vi "export example information.vi"() -> ()   [LabVIEW 2020]
uses:
  <vilib>/JDP Science/JSONtext/LVClass Serializer/JSONtext LVClass Serializer.lvclass
  4edb9a30-9a21-4ee1-8258-10869d222808.vi
  <vilib>/Utility/NIReport.llb/NI_ReportGenerationCore.lvlib
panel:
  out "error out":errorcluster
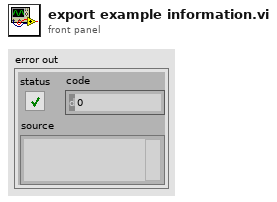
[diagram p1: front panel]
types:
  T1 = enum16{"open", "replace", "create", "open or create", "replace or create", "replace or create with confirmation"}
  T2 = cluster{"Printing:Custom All Controls?":bool, "Printing:Custom Connector?":bool, "Printing:Custom Control Descriptions?":bool, "Printing:Custom Control Types?":bool, "Printing:Custom Controls?":bool, "Printing:Custom Description?":bool, "Printing:Custom Diagram Hidden?":bool, "Printing:Custom Diagram Repeat?":bool, "Printing:Custom Diagram?":bool, "Printing:Custom Hierarchy?":bool, "Printing:Custom History?":bool, "Printing:Custom Panel Border?":bool, "Printing:Custom Panel?":bool, "Printing:Custom SubVIs?":bool}
  T3 = cluster{"vi name":string, "diagram image":path, "description":string}
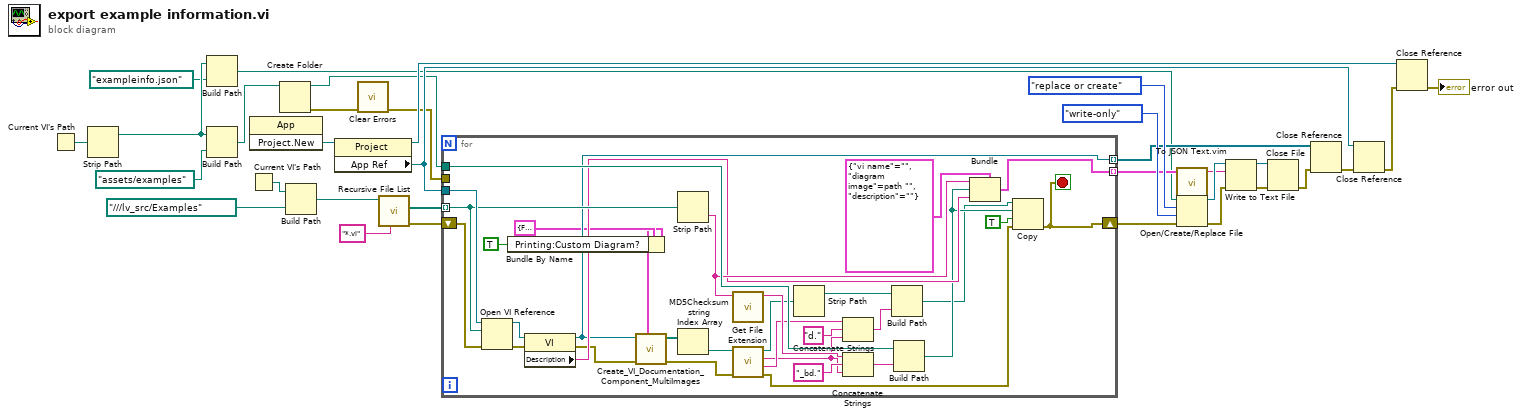
[diagram p0: block diagram]
diagram:
  n1 = Current VI's Path() -> (path=w30:path)
  n2 = Strip Path(path=w30) -> (stripped path=w3:path)  [unwired: 1 out]
  n3 = Build Path(base path=w3, name or relative path=path "exampleinfo.json") -> (appended path=w1:path)
  n4 = Build Path(base path=w3, name or relative path=path "assets/examples") -> (appended path=w9:path)
  n5 = Current VI's Path() -> (path=w32:path)
  n6 = invoke class="App" method="Project.New"() -> ("Project:New"=w25:refnum<vi>)  [unwired: 3 in, 2 out]
  n7 = Create Folder(path (use dialog)=w9) -> (created path=w7:path, error out=w28:errorcluster)  [unwired: 2 in, 1 out]
  n8 = Build Path(base path=w32, name or relative path=path "../../../lv_src/Examples") -> (appended path=w27:path)
  n9 = property class="Project"(reference=w25) -> (reference out=w22:refnum<vi>, "App Ref"=w20:refnum<vi>)  [unwired: 1 in, 1 out]
  n10 = call <vilib>:"Clear Errors.vi"("error in (no error)"=w28) -> ("error out"=w8:errorcluster)  [unwired: 5 in, 1 out]
  n11 = call <vilib>:"Recursive File List.vi"("pattern"="*.vi", "Folder Path"=w27) -> ("error out"=w6:errorcluster, "All Files in Dir"=w19:path[])  [unwired: 5 in, 3 out]
  n12 = for {
    tunnel: w20 -> [w64]
    tunnel: w19 -> [w62] mode=indexing
    tunnel: [w51] -> w10 mode=indexing
    tunnel: w8 -> [_]
    tunnel: w7 -> [w61]
    shift-right: [w37] -> w5
    shift-left: w6 -> [w58]
    tunnel: [w53] -> w4 mode=indexing
    stop <- w37 stop-if-true
    n13 = Open VI Reference(application reference (local)=w64, vi path=w62, error in (no error)=w58) -> (vi reference=w55:refnum<vi>, error out=w63:errorcluster)  [unwired: 3 in]
    n14 = Bundle By Name(cluster=T2 {"Printing:Custom All Controls?"=FALSE, "Printing:Custom Connector?"=FALSE, "Printing:Custom Control Descriptions?"=FALSE, "Printing:Custom Control Types?"=FALSE, "Printing:Custom Controls?"=FALSE, "Printing:Custom Description?"=FALSE, "Printing:Custom Diagram Hidden?"=FALSE, "Printing:Custom Diagram Repeat?"=FALSE, "Printing:Custom Diagram?"=TRUE, "Printing:Custom Hierarchy?"=FALSE, "Printing:Custom History?"=FALSE, "Printing:Custom Panel Border?"=FALSE, "Printing:Custom Panel?"=FALSE, "Printing:Custom SubVIs?"=FALSE} ("Content Options"), "Printing:Custom Diagram?"=TRUE) -> (w34:T2)
    n15 = property class="VI"(reference=w55, error in=w63) -> (reference out=w51:refnum<vi>, error out=w50:errorcluster, "Description"=w54:string)
    n16 = call <vilib>:"Create_VI_Documentation_Component_MultiImages.vi"("Content Options"=w34, "error in (no error)"=w50, "VI"=w51) -> ("error out"=w49:errorcluster, "Paths to images"=w47:path[])  [unwired: 7 in]
    n17 = Strip Path(path=w62) -> (name=w56:string)  [unwired: 1 out]
    n18 = Index Array(array=w47) -> (element=w43:path)  [unwired: 1 in]
    n19 = call "MD5Checksum string.vi"("Message String"=w56) -> ("MD5 message-digest"=w60:string)  [unwired: 10 in]
    n20 = call <vilib>:"Get File Extension.vi"("error in (no error)"=w49, "file"=w43) -> ("error out"=w44:errorcluster, "filename without extension"=w36:string, "lowercase file extension"=w35:string, "dup file"=w42:path)  [unwired: 5 in, 1 out]
    n21 = Strip Path(path=w42) -> (stripped path=w41:path)  [unwired: 1 out]
    n22 = Concatenate Strings(w36, "d." ("string"), w35) -> (w38:string)
    n23 = Concatenate Strings(w60, "_bd." ("string"), w35) -> (w59:string)
    n24 = Build Path(base path=w41, name or relative path=w38) -> (appended path=w40:path)
    n25 = Build Path(base path=w61, name or relative path=w59) -> (appended path=w46:path)
    n26 = Bundle(cluster=T3 {"vi name"="", "diagram image"=path "", "description"=""}, "vi name"=w56, "diagram image"=w46, "description"=w54) -> (w53:T3)
    n27 = Copy(8:w44, 9:TRUE ("overwrite (F)"), 10:w46, 11:w40) -> (0:w37:errorcluster)  [unwired: 1 in, 2 out]
  }
  n28 = call "To JSON Text.vim"("Anything"=w4) -> ("<JSON>"=w12:string)  [unwired: 9 in, 1 out]
  n29 = Open/Create/Replace File(file path (use dialog)=w1, error in=w5, operation (0:open)=T1."replace or create", access (0:read/write)=enum16{"read/write", "read-only", "write-only"}."write-only") -> (refnum out=w15:refnum<file>, error out=w16:errorcluster)  [unwired: 2 in, 1 out]
  n30 = Write to Text File(file (use dialog)=w15, text=w12, error in=w16) -> (refnum out=w17:refnum<file>, error out=w18:errorcluster)  [unwired: 1 in, 1 out]
  n31 = Close File(refnum=w17, error in=w18) -> (error out=w11:errorcluster)  [unwired: 1 out]
  n32 = Close Reference(reference=w10, error in (no error)=w11) -> (error out=w21:errorcluster)
  n33 = Close Reference(reference=w20, error in (no error)=w21) -> (error out=w24:errorcluster)
  n34 = Close Reference(reference=w22, error in (no error)=w24) -> (error out=→"error out":errorcluster)
